vi "is cancelled.vi"(11 "null task token in":refnum<class "null task token.lvclass">) -> (2 "cancelled?":bool, 3 "null task token out":refnum<class "null task token.lvclass">)   [LabVIEW 2013, in "null task token.lvclass"]
uses:
  null task token.lvclass
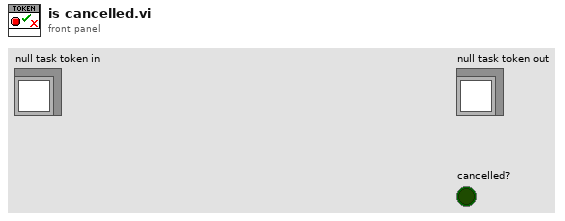
[diagram p1: front panel]
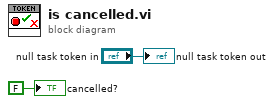
[diagram p0: block diagram]
diagram:
  "null task token out" <- "null task token in"
  "cancelled?" <- FALSE ("cancelled?")
